vi "Is Variant Type Numeric.vi"(8 "error in (no error)":errorcluster, 11 "variant":variant) -> (0 "error out":errorcluster, 2 "Type":T1=enum."Boolean", 3 "Is numeric?":bool)   [LabVIEW 2020, in "RxnRover.lvlib"]
doc: "Check if the variant contents are a numeric type."
uses:
  RxnRover.lvlib
  Supported Parameter Variant Types.ctl
  <vilib>/Utility/Data Type/NI_Data Type.lvlib
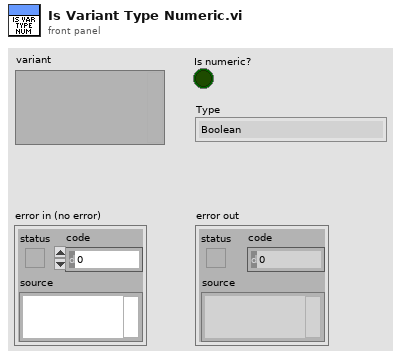
[diagram p1: front panel]
types:
  T1 = typedef "RxnRover.lvlib/Supported Parameter Variant Types.ctl" = enum16{"Unsupported", "Numeric", "Boolean", "String", "Path"}
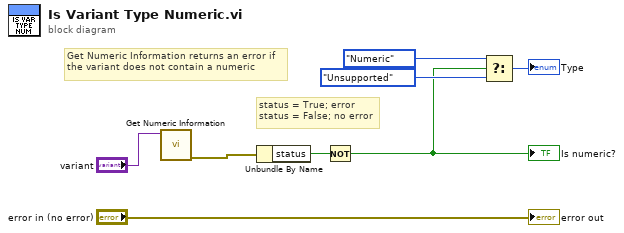
[diagram p0: block diagram]
diagram:
  # "Get Numeric Information returns an error if the variant does not contain a numeric"
  # "status = True; error\nstatus = False; no error"
  n1 = call <vilib>:"Get Numeric Information.vi"("variant"="variant") -> ("error out"=w7:errorcluster)  [unwired: 7 in, 3 out]
  n2 = Unbundle By Name(w7) -> ("status"=w6:bool)
  n3 = Not(x=w6) -> (.not. x?=w1:bool)
  "Is numeric?" <- w1
  n4 = Select(t=Supported_Parameter_Variant_Types."Numeric" ("Supported Parameter Variant Types"), s=w1, f=Supported_Parameter_Variant_Types."Unsupported" ("Supported Parameter Variant Types")) -> (s? t:f=→"Type":T1)
  "error out" <- "error in (no error)"
